vi "בדיקת מפל מתח בין הדקי הממסר תחת עומס 5.vi"(8 "error":errorcluster, 10 "lines":tag="PXI1Slot8/port0/line1", 11 "Path for Log":path) -> (0 "error IO":errorcluster, 1 "בטוח כן/לא":bool, 2 "מפל מתח בין דקי הממסר תחת עומס":dbl, 3 "תוצאה זמנית":dbl)   [LabVIEW 2014]
uses:
  M9700 Driver/85/vi.lib/M9700 Modbus.llb/CTL Register Address.ctl
  M9700 Driver/86/vi.lib/M9700 Modbus.llb/CTL CMD Register.ctl
  <vilib>/Instr/_visa.llb/VISA Configure Serial Port (Instr).vi
  <vilib>/DAQmx/create/channels.llb/DAQmx Create Channel (DO-Digital Output).vi
  <vilib>/DAQmx/write.llb/DAQmx Write (Digital Bool 1Line 1Point).vi
panel:
  out "progress":dbl(slide) min=0.0 max=10.0 scale=0.0..10.0
  in  "stop":bool
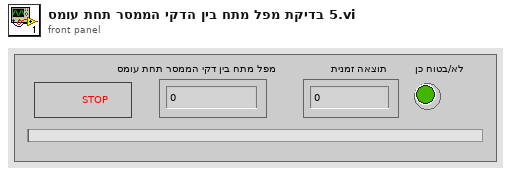
[diagram p1: front panel]
types:
  T1 = enum32{"Invalid", "Standard", "Closed", "Hidden", "Minimized", "Maximized"}
  T2 = typedef "CTL CMD Register.ctl" = u8
  T3 = typedef "CTL Register Address.ctl" = u16
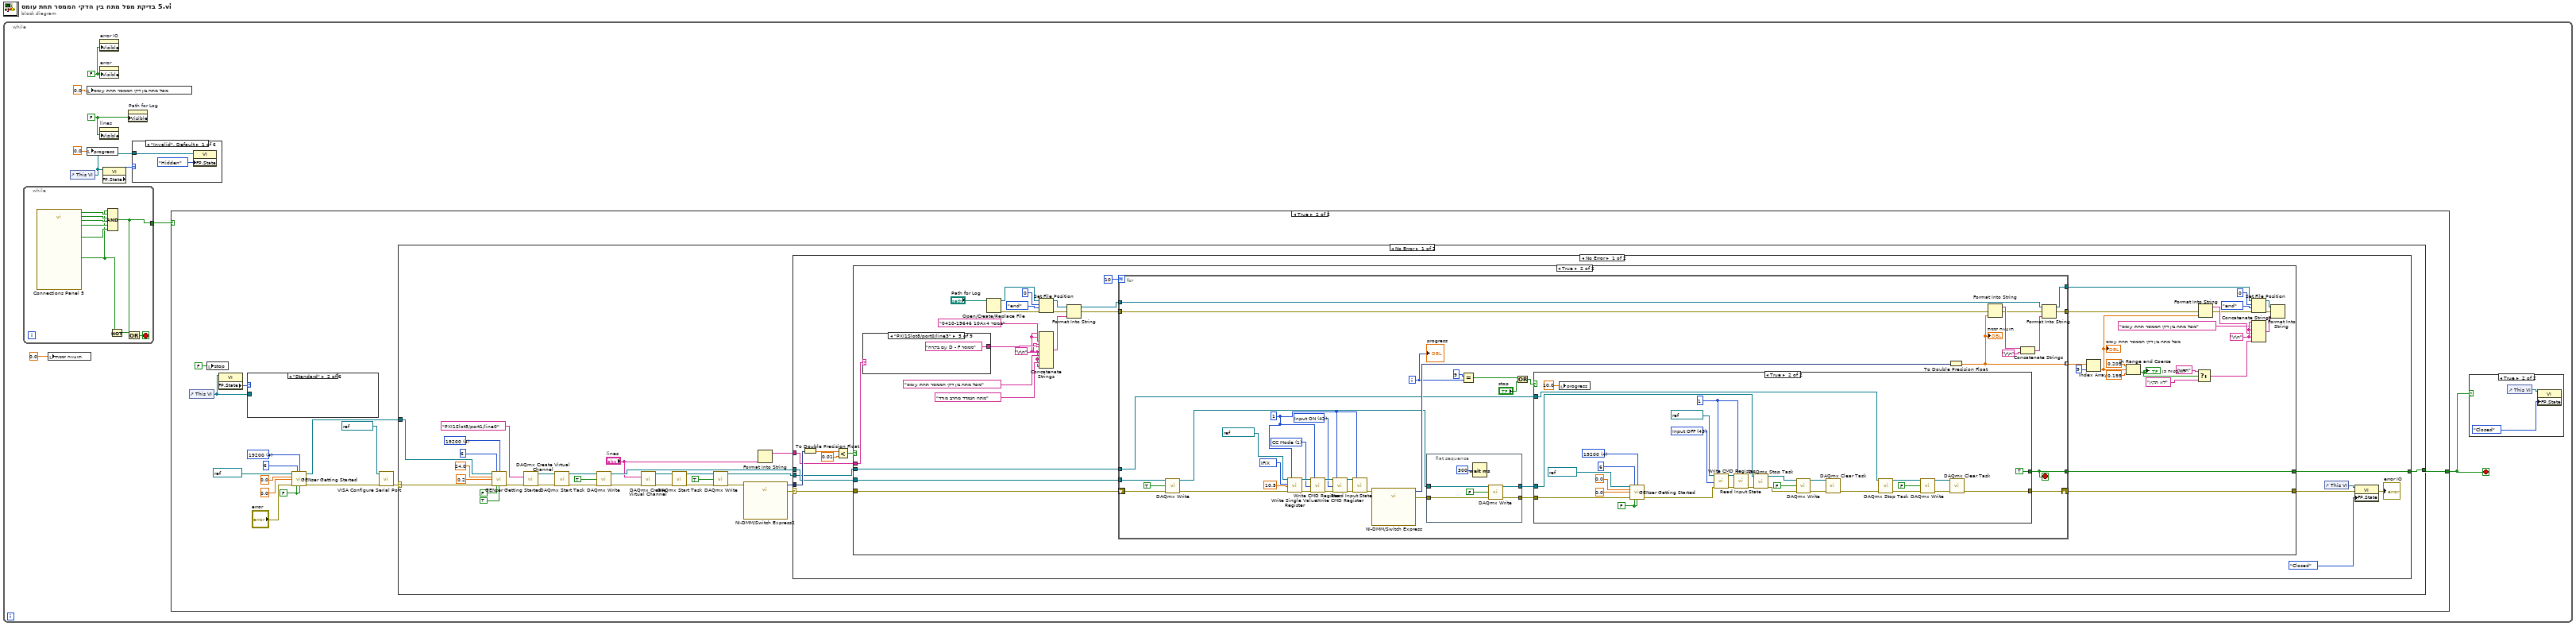
[diagram p0: block diagram]
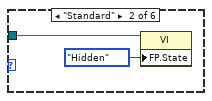
[diagram p2: hidden frame]
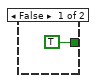
[diagram p8: hidden frame]
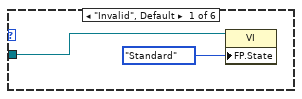
[diagram p9: hidden frame]
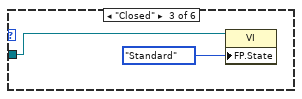
[diagram p10: hidden frame]
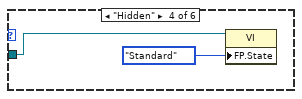
[diagram p11: hidden frame]
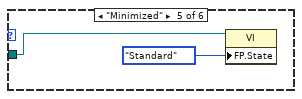
[diagram p12: hidden frame]
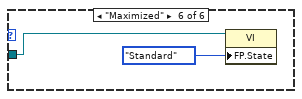
[diagram p13: hidden frame]
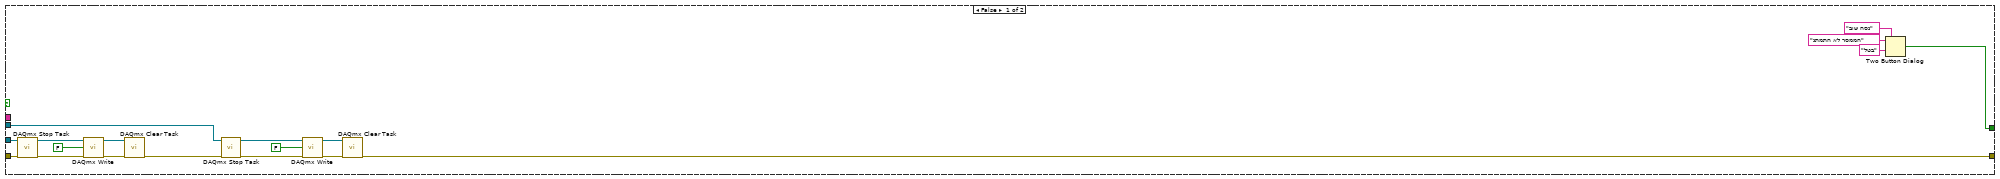
[diagram p14: hidden frame]
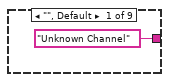
[diagram p15: hidden frame]
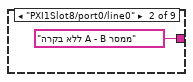
[diagram p16: hidden frame]
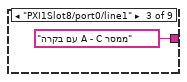
[diagram p17: hidden frame]
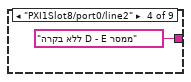
[diagram p18: hidden frame]
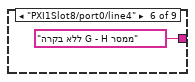
[diagram p19: hidden frame]
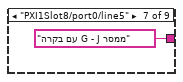
[diagram p20: hidden frame]
diagram:
  n1 = while {
    stop <- w3 stop-if-true
    w4 = FALSE ("Visible")
    w5 = FALSE ("Visible")
    n2 = while {
      tunnel: [w10] -> w9
      stop <- w13 stop-if-true
      n3 = call "Connections Panel 5.vi"() -> ("Input Name 10"=w14:bool, "Input Name 6"=w18:bool, "Input Name 7"=w17:bool, "Input Name 8"=w16:bool, "Input Name 9"=w15:bool, "OK"=w11:bool)  [unwired: 13 in, 1 out]
      n4 = Compound Arithmetic op=AND(w11, w18, w17, w16, w15, w14) -> (w10:bool)
      n5 = Not(x=w11) -> (.not. x?=w12:bool)
      n6 = Or(x=w12, y=w10) -> (x .or. y?=w13:bool)
    }
    n7 = local write "תוצאה זמנית"(0.0 ("תוצאה זמנית")) -> ()
    n8 = control-ref of="This VI"() -> (w2:refnum<vi>)
    n9 = local write "מפל מתח בין דקי הממסר תחת עומס"(0.0 ("מפל מתח בין דקי הממסר תחת עומס")) -> ()
    n10 = local write "progress"(0.0 ("progress")) -> ()
    n11 = property on="error IO" class="Clust (strict)"("Visible"=w5) -> ()  [unwired: 2 in, 2 out]
    n12 = property on="error" class="Clust (strict)"("Visible"=w5) -> ()  [unwired: 2 in, 2 out]
    n13 = property on="lines" class="DAQmxName"("Visible"=w4) -> ()  [unwired: 2 in, 2 out]
    n14 = property class="VI"(reference=w2) -> ("FP.State"=w1:T1)  [unwired: 1 in, 2 out]
    n15 = property on="Path for Log" class="Path"("Visible"=w4) -> ()  [unwired: 2 in, 2 out]
    n16 = case shown="\"Invalid\", Default" w1 {
      tunnel: w2 -> [w19 w21 _ _ _ _]
      frame "Invalid", Default {
        n17 = property class="VI"(reference=w19, "FP.State"=T1."Hidden" ("Front Panel Window:State")) -> ()  [unwired: 1 in, 2 out]
      }
      frame "Standard" {
        n18 = property class="VI"(reference=w21, "FP.State"=T1."Hidden" ("Front Panel Window:State")) -> ()  [unwired: 1 in, 2 out]
      }
      frame "Closed" {
      }
      frame "Hidden" {
      }
      frame "Minimized" {
      }
      frame "Maximized" {
      }
    }
    n19 = case shown="True" w9 {
      tunnel: [TRUE w26] -> w3
      frame False {
      }
      frame True {
        w31 = FALSE ("Output On (T)")
        w37 = u16 4 items=["1200", "2400", "4800", "9600", "19200"] ("BAUD")
        n20 = control-ref of="This VI"() -> (w28:refnum<vi>)
        n21 = local write "stop"(FALSE ("stop")) -> ()
        n22 = property class="VI"(reference=w28) -> ("FP.State"=w29:T1)  [unwired: 1 in, 2 out]
        n23 = case shown="\"Standard\"" w29 {
          tunnel: w28 -> [w41 _ w43 w45 w47 w49]
          frame "Invalid", Default {
            n24 = property class="VI"(reference=w41, "FP.State"=T1."Standard" ("Front Panel Window:State")) -> ()  [unwired: 1 in, 2 out]
          }
          frame "Standard" {
          }
          frame "Closed" {
            n25 = property class="VI"(reference=w43, "FP.State"=T1."Standard" ("Front Panel Window:State")) -> ()  [unwired: 1 in, 2 out]
          }
          frame "Hidden" {
            n26 = property class="VI"(reference=w45, "FP.State"=T1."Standard" ("Front Panel Window:State")) -> ()  [unwired: 1 in, 2 out]
          }
          frame "Minimized" {
            n27 = property class="VI"(reference=w47, "FP.State"=T1."Standard" ("Front Panel Window:State")) -> ()  [unwired: 1 in, 2 out]
          }
          frame "Maximized" {
            n28 = property class="VI"(reference=w49, "FP.State"=T1."Standard" ("Front Panel Window:State")) -> ()  [unwired: 1 in, 2 out]
          }
        }
        n29 = call "GENser Getting Started.vi"("VISA"=refnum<visa-resource-name> "COM6", "GEN Addr"=i16 6, "BAUD"=w37, "Voltage Limit"=0.0, "Current Limit"=0.0, "error"="error", "Reset (T)"=w31, "Output On (T)"=w31) -> ("VISA out"=w39:refnum<visa-resource-name>, "error out"=w27:errorcluster)  [unwired: 4 in, 2 out]
        n30 = call-poly "VISA Configure Serial Port"("VISA resource name"=refnum<visa-resource-name> "COM13", "error in (no error)"=w27) -> ("error out"=w32:errorcluster)  [unwired: 4 in, 9 out]
        n31 = case shown="No Error" w32 {
          selector: w32 -> [w76 _]
          tunnel: w39 -> [w79 _]
          tunnel: [w78 w245] -> w26
          frame No Error {
            w70 = u16 4 items=["1200", "2400", "4800", "9600", "19200"] ("BAUD")
            n32 = call "GENser Getting Started.vi"("VISA"=w79, "GEN Addr"=i16 6, "BAUD"=w70, "Voltage Limit"=24.0, "Current Limit"=0.2, "error"=w76, "Reset (T)"=FALSE, "Output On (T)"=TRUE) -> ("error out"=w64:errorcluster)  [unwired: 4 in, 3 out]
            n33 = call-poly <vilib>:"DAQmx Create Virtual Channel.vi"("lines"=tag "PXI1Slot5/port1/line0", "error in"=w64) -> ("task out"=w60:refnum<k21>, "error out"=w61:errorcluster)  [unwired: 12 in]
            n34 = call <vilib>:"DAQmx Start Task.vi"("task/channels in"=w60, "error in"=w61) -> ("task out"=w58:refnum<k21>, "error out"=w57:errorcluster)  [unwired: 12 in]
            n35 = call-poly <vilib>:"DAQmx Write.vi"("task/channels in"=w58, "data"=TRUE, "error in"=w57) -> ("task out"=w68:refnum<k21>, "error out"=w67:errorcluster)  [unwired: 10 in, 1 out]
            n36 = call-poly <vilib>:"DAQmx Create Virtual Channel.vi"("lines"="lines", "error in"=w67) -> ("task out"=w51:refnum<k21>, "error out"=w52:errorcluster)  [unwired: 12 in]
            n37 = call <vilib>:"DAQmx Start Task.vi"("task/channels in"=w51, "error in"=w52) -> ("task out"=w54:refnum<k21>, "error out"=w53:errorcluster)  [unwired: 12 in]
            n38 = call-poly <vilib>:"DAQmx Write.vi"("task/channels in"=w54, "data"=TRUE, "error in"=w53) -> ("task out"=w66:refnum<k21>, "error out"=w63:errorcluster)  [unwired: 10 in, 1 out]
            n39 = call "NI-DMM/Switch Express2"("error in"=w63) -> ("signals out"=w77:dynamicdata, "error out"=w62:errorcluster)  [unwired: 16 in, 1 out]
            n40 = Format Into String("lines") -> (resulting string=w69:string)  [unwired: 3 in, 1 out]
            n41 = case shown="No Error" w62 {
              selector: w62 -> [w90 _]
              tunnel: [w89 w240] -> w78
              tunnel: w77 -> [w92 _]
              tunnel: w68 -> [w83 _]
              tunnel: w69 -> [w81 _]
              tunnel: w66 -> [w80 _]
              frame No Error {
                n42 = To Double Precision Float(number=w92) -> (double precision float=w88:dbl)
                n43 = Less?(x=w88, y=0.01) -> (x < y?=w91:bool)
                n44 = case shown="True" w91 {
                  tunnel: w90 -> [w100 w114]
                  tunnel: [w93 w152] -> w89
                  tunnel: [w97 w146] -> w84
                  tunnel: w83 -> [w99 w147]
                  tunnel: w81 -> [_ w116]
                  tunnel: w80 -> [w98 w115]
                  frame False {
                    n45 = call <vilib>:"DAQmx Stop Task.vi"("task/channels in"=w99, "error in"=w100) -> ("task out"=w111:refnum<k21>, "error out"=w109:errorcluster)  [unwired: 12 in]
                    n46 = call-poly <vilib>:"DAQmx Write.vi"("task/channels in"=w111, "data"=FALSE, "error in"=w109) -> ("task out"=w108:refnum<k21>, "error out"=w107:errorcluster)  [unwired: 10 in, 1 out]
                    n47 = call <vilib>:"DAQmx Clear Task.vi"("task in"=w108, "error in"=w107) -> ("error out"=w101:errorcluster)  [unwired: 13 in]
                    n48 = call <vilib>:"DAQmx Stop Task.vi"("task/channels in"=w98, "error in"=w101) -> ("task out"=w106:refnum<k21>, "error out"=w104:errorcluster)  [unwired: 12 in]
                    n49 = call-poly <vilib>:"DAQmx Write.vi"("task/channels in"=w106, "data"=FALSE, "error in"=w104) -> ("task out"=w103:refnum<k21>, "error out"=w102:errorcluster)  [unwired: 10 in, 1 out]
                    n50 = call <vilib>:"DAQmx Clear Task.vi"("task in"=w103, "error in"=w102) -> ("error out"=w97:errorcluster)  [unwired: 13 in]
                    n51 = Two Button Dialog(message="הממסר לא התמתג", 1:"נסה שוב" ("F button name (\"Cancel\")"), 2:"בטל" ("T button name (\"OK\")")) -> (T button?=w93:bool)
                  }
                  frame True {
                    w133 = "\r\n"
                    w112 = "\r\n"
                    n52 = case shown="\"PXI1Slot8/port0/line3\"" w116 {
                      tunnel: ["Unknown Channel" "ללא בקרה A - B ממסר" "עם בקרה A - C ממסר" "ללא בקרה D - E ממסר" "עם בקרה D - F ממסר" "ללא בקרה G - H ממסר" "עם בקרה G - J ממסר" "ללא בקרה P - N ממסר" "עם בקרה P - L ממסר"] -> w113
                      frame "", Default {
                      }
                      frame "PXI1Slot8/port0/line0" {
                      }
                      frame "PXI1Slot8/port0/line1" {
                      }
                      frame "PXI1Slot8/port0/line2" {
                      }
                      frame "PXI1Slot8/port0/line3" {
                      }
                      frame "PXI1Slot8/port0/line4" {
                      }
                      frame "PXI1Slot8/port0/line5" {
                      }
                      frame "PXI1Slot8/port0/line6" {
                      }
                      frame "PXI1Slot8/port0/line7" {
                      }
                    }
                    n53 = Open/Create/Replace File(file path (use dialog)="Path for Log") -> (refnum out=w143:refnum<file>, error out=w142:errorcluster)  [unwired: 5 in, 1 out]
                    n54 = Set File Position(offset (in bytes) (0)=i64 0, refnum=w143, from (0:start)=enum16{"start", "end", "current"}."end", error in=w142) -> (refnum out=w139:refnum<file>, error out=w136:errorcluster)
                    n55 = Concatenate Strings(w112, w112, "0410-19646 10Ax4 ממסר", w112, w113, w112, "מפל מתח בין דקי הממסר תחת עומס", w112, "מתח הנמדד מהרב מודד", w112) -> (w141:string)
                    n56 = Format Into String(initial string=w139, error in=w136, w141) -> (resulting string=w134:refnum<file>, error out=w135:errorcluster)  [unwired: 1 in]
                    n57 = for {
                      N: 10 -> [_]
                      tunnel: [w184] -> w152
                      shift-right: [w182] -> w146
                      shift-left: w114 -> [w177]
                      tunnel: [w164] -> w151 mode=indexing
                      tunnel: w147 -> [w178]
                      tunnel: w135 -> [w168]
                      tunnel: w134 -> [w170]
                      tunnel: [w167] -> w127
                      tunnel: [w166] -> w118
                      tunnel: w115 -> [w165]
                      i -> [w181]
                      stop <- w184 stop-if-true
                      w192 = T2 42 items=["CC Mode"=1, "CV Mode"=2, "CW Mode"=3, "CR Mode"=4, "Short Mode"=26, "Set SysPara"=41, "Input ON"=42, "Input OFF"=43] ("CMD Register Value")
                      w195 = u8 1 ("Load Address")
                      w198 = T2 1 items=["CC Mode"=1, "CV Mode"=2, "CW Mode"=3, "CR Mode"=4, "Short Mode"=26, "Set SysPara"=41, "Input ON"=42, "Input OFF"=43] ("CMD Register Value")
                      w201 = T3 2561 items=["REMOTE"=1283, "ISTATE"=1296, "CMD"=2560, "IFIX"=2561, "UFIX"=2563, "PFIX"=2565, "RFIX"=2567, "IMAX"=2612, "UMAX"=2614, "PMAX"=2616, "U"=2816, "I"=2818, "MODEL"=2822, "EDITION"=2823] ("Register Address")
                      n58 = call-poly <vilib>:"DAQmx Write.vi"("task/channels in"=w178, "data"=TRUE, "error in"=w177) -> ("task out"=w176:refnum<k21>, "error out"=w163:errorcluster)  [unwired: 10 in, 1 out]
                      n59 = call "Write Single Value Register.vi"("VISA resource name"=refnum<visa-resource-name> "COM13", "Starting Address(HEX)"=w201, "Register Single Value"=sgl 10.5, "error in"=w163, "Load Address"=w195) -> ("VISA resource name out"=w200:refnum<visa-resource-name>, "error out"=w199:errorcluster)  [unwired: 13 out]
                      n60 = call "Write CMD Register.vi"("VISA resource name"=w200, "CMD Value"=w198, "error in"=w199, "Load Address"=w195) -> ("VISA resource name out"=w196:refnum<visa-resource-name>, "error out"=w193:errorcluster)  [unwired: 14 out]
                      n61 = call "Write CMD Register.vi"("VISA resource name"=w196, "CMD Value"=w192, "error in"=w193, "Load Address"=w195) -> ("VISA resource name out"=w194:refnum<visa-resource-name>, "error out"=w191:errorcluster)  [unwired: 14 out]
                      n62 = call "Read Input State.vi"("VISA resource name"=w194, "error in"=w191, "Load Address"=w195) -> ("error out"=w190:errorcluster)  [unwired: 16 out]
                      n63 = call "NI-DMM/Switch Express"("error in"=w190) -> ("signals out"=w189:dynamicdata, "error out"=w179:errorcluster)  [unwired: 16 in, 1 out]
                      n64 = flat-sequence {
                        tunnel: [w207] -> w180
                        tunnel: w179 -> [w206]
                        tunnel: w176 -> [w204]
                        tunnel: [w203] -> w174
                        frame #0 {
                          n65 = Wait (ms)(milliseconds to wait=u32 300) -> ()  [unwired: 1 out]
                          n66 = call-poly <vilib>:"DAQmx Write.vi"("task/channels in"=w204, "data"=FALSE, "error in"=w206) -> ("task out"=w203:refnum<k21>, "error out"=w207:errorcluster)  [unwired: 10 in, 1 out]
                        }
                      }
                      n67 = Equal?(x=9, y=w181) -> (x = y?=w186:bool)
                      n68 = Or(x=w186, y="stop") -> (x .or. y?=w187:bool)
                      n69 = case shown="True" w187 {
                        tunnel: [FALSE TRUE] -> w184
                        tunnel: w180 -> [w208 w233]
                        tunnel: [w208 w213] -> w182
                        tunnel: w174 -> [_ w219]
                        tunnel: w165 -> [_ w211]
                        frame False {
                        }
                        frame True {
                          w227 = u8 1 ("Load Address")
                          w230 = T2 43 items=["CC Mode"=1, "CV Mode"=2, "CW Mode"=3, "CR Mode"=4, "Short Mode"=26, "Set SysPara"=41, "Input ON"=42, "Input OFF"=43] ("CMD Register Value")
                          w232 = FALSE ("Reset (T)")
                          w235 = u16 4 items=["1200", "2400", "4800", "9600", "19200"] ("BAUD")
                          n70 = local write "progress"(10.0 ("progress")) -> ()
                          n71 = call "GENser Getting Started.vi"("VISA"=refnum<visa-resource-name> "COM6", "GEN Addr"=i16 6, "BAUD"=w235, "Voltage Limit"=0.0, "Current Limit"=0.0, "error"=w233, "Reset (T)"=w232, "Output On (T)"=w232) -> ("error out"=w210:errorcluster)  [unwired: 4 in, 3 out]
                          n72 = call "Write CMD Register.vi"("VISA resource name"=refnum<visa-resource-name> "COM13", "CMD Value"=w230, "error in"=w210, "Load Address"=w227) -> ("VISA resource name out"=w228:refnum<visa-resource-name>, "error out"=w231:errorcluster)  [unwired: 14 out]
                          n73 = call "Read Input State.vi"("VISA resource name"=w228, "error in"=w231, "Load Address"=w227) -> ("error out"=w220:errorcluster)  [unwired: 16 out]
                          n74 = call <vilib>:"DAQmx Stop Task.vi"("task/channels in"=w219, "error in"=w220) -> ("task out"=w225:refnum<k21>, "error out"=w223:errorcluster)  [unwired: 12 in]
                          n75 = call-poly <vilib>:"DAQmx Write.vi"("task/channels in"=w225, "data"=FALSE, "error in"=w223) -> ("task out"=w222:refnum<k21>, "error out"=w221:errorcluster)  [unwired: 10 in, 1 out]
                          n76 = call <vilib>:"DAQmx Clear Task.vi"("task in"=w222, "error in"=w221) -> ("error out"=w212:errorcluster)  [unwired: 13 in]
                          n77 = call <vilib>:"DAQmx Stop Task.vi"("task/channels in"=w211, "error in"=w212) -> ("task out"=w218:refnum<k21>, "error out"=w216:errorcluster)  [unwired: 12 in]
                          n78 = call-poly <vilib>:"DAQmx Write.vi"("task/channels in"=w218, "data"=FALSE, "error in"=w216) -> ("task out"=w215:refnum<k21>, "error out"=w214:errorcluster)  [unwired: 10 in, 1 out]
                          n79 = call <vilib>:"DAQmx Clear Task.vi"("task in"=w215, "error in"=w214) -> ("error out"=w213:errorcluster)  [unwired: 13 in]
                        }
                      }
                      n80 = To Double Precision Float(number=w189) -> (double precision float=w164:dbl)
                      "תוצאה זמנית" <- w164
                      n81 = Format Into String(error in=w168, w164) -> (resulting string=w172:string, error out=w169:errorcluster)  [unwired: 2 in]
                      n82 = Concatenate Strings(w172, "\r\n") -> (w171:string)
                      n83 = Format Into String(initial string=w170, error in=w169, w171) -> (resulting string=w167:refnum<file>, error out=w166:errorcluster)  [unwired: 1 in]
                      "progress" <- w181
                    }
                    n84 = Index Array(array=w151, index=9) -> (element=w126:dbl)
                    "מפל מתח בין דקי הממסר תחת עומס" <- w126
                    n85 = In Range and Coerce(upper limit=0.205, x=w126, lower limit=0.195) -> (In Range?=w121:bool)  [unwired: 1 out]
                    "בטוח כן/לא" <- w121
                    n86 = Select(t="תקין", s=w121, f="לא תקין") -> (s? t:f=w120:string)
                    n87 = Format Into String(error in=w118, w126) -> (resulting string=w125:string, error out=w119:errorcluster)  [unwired: 2 in]
                    n88 = Set File Position(offset (in bytes) (0)=i64 0, refnum=w127, from (0:start)=enum16{"start", "end", "current"}."end", error in=w119) -> (refnum out=w130:refnum<file>, error out=w129:errorcluster)
                    n89 = Concatenate Strings(w133, "מפל מתח בין דקי הממסר תחת עומס" ("string"), w133, w125, w133, w120) -> (w128:string)
                    n90 = Format Into String(initial string=w130, error in=w129, w128) -> ()  [unwired: 1 in, 2 out]
                  }
                }
                n91 = control-ref of="This VI"() -> (w86:refnum<vi>)
                n92 = property class="VI"(reference=w86, error in=w84, "FP.State"=T1."Closed" ("Front Panel Window:State")) -> (error out=→"error IO":errorcluster)  [unwired: 1 out]
              }
              frame Error {
                n93 = Two Button Dialog(message="בעיית דגימת נתונים ע\"י הכרטיס רב מודד", 1:"ביטול" ("F button name (\"Cancel\")"), 2:"נסה שוב" ("T button name (\"OK\")")) -> (T button?=w241:bool)
                n94 = Not(x=w241) -> (.not. x?=w240:bool)
              }
            }
          }
          frame Error {
            n95 = Two Button Dialog(message="בעיית תקשורת עם ספק קוח", 1:"ביטול" ("F button name (\"Cancel\")"), 2:"נסה שוב" ("T button name (\"OK\")")) -> (T button?=w246:bool)
            n96 = Not(x=w246) -> (.not. x?=w245:bool)
          }
        }
      }
    }
    n97 = case shown="True" w3 {
      frame False {
      }
      frame True {
        n98 = control-ref of="This VI"() -> (w24:refnum<vi>)
        n99 = property class="VI"(reference=w24, "FP.State"=T1."Closed" ("Front Panel Window:State")) -> ()  [unwired: 1 in, 2 out]
      }
    }
  }
